vi "UserVars-Get Bernoulli Function.vi"(0 "Expr in":string, 11 "error in (no error)":errorcluster) -> (6 "X":dbl[](array[numeric]), 8 "PDF":dbl[](array[numeric]), 10 "Ref Pts":dbl[](array[numeric]), 15 "error out":errorcluster)   [LabVIEW 2020]
uses:
  <vilib>/Analysis/1siggen.llb/Ramp Pattern by Samples.vi
  <vilib>/regexp/Match Regular Expression.xnode
  <vilib>/Analysis/NI_AALBase.lvlib
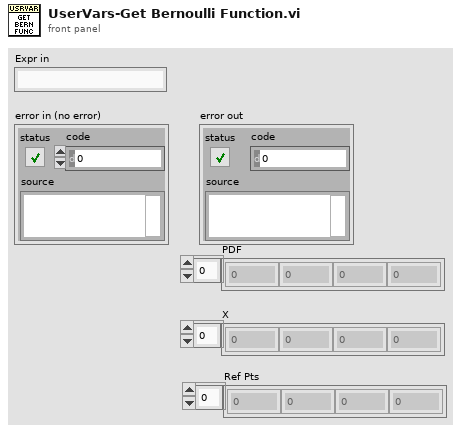
[diagram p1: front panel]
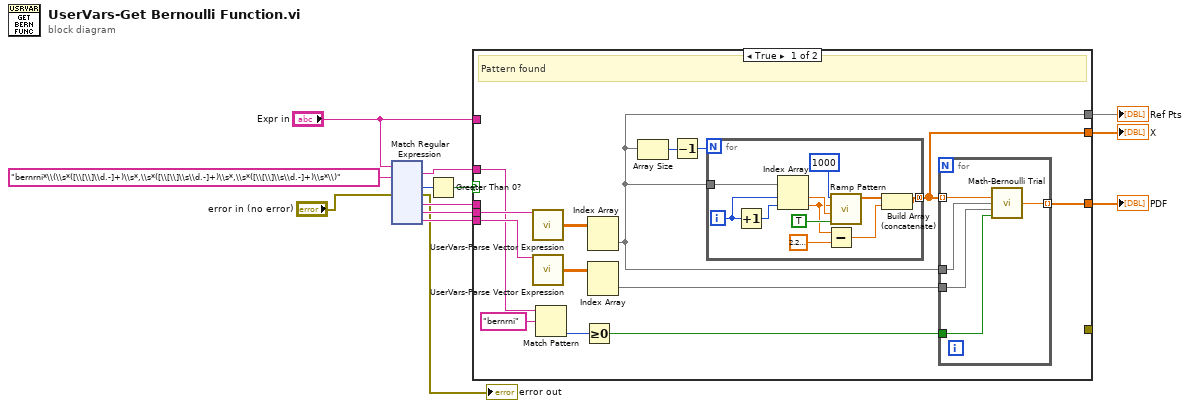
[diagram p0: block diagram]
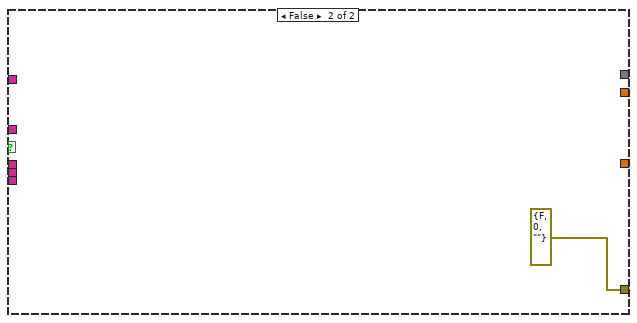
[diagram p2: hidden frame]
diagram:
  n1 = xnode "Match Regular Expression"("input string"="Expr in", "regular expression"="bernrni*\\(\\s*([\\[\\]\\d.-]+)\\s*,\\s*([\\[\\]\\s\\d.-]+)\\s*,\\s*([\\[\\]\\s\\d.-]+)\\s*\\)" ("String"), "error in"="error in (no error)") -> ("whole match"=w10:string, "offset past match"=w11:i32, "error out"=→"error out":errorcluster, "submatch 1"=w9:string, "submatch 2"=w8:string, "submatch 3"=w6:string)  [unwired: 3 in, 2 out]
  n2 = Greater Than 0?(x=w11) -> (x > 0?=w7:bool)
  n3 = case shown="True" w7 {
    tunnel: "Expr in" -> [_ _]
    tunnel: w10 -> [w17 _]
    tunnel: w9 -> [_ _]
    tunnel: w8 -> [w27 _]
    tunnel: w6 -> [w26 _]
    tunnel: [w20 _] -> w4
    tunnel: [_ errorcluster {"status"=FALSE, "code"=0, "source"=""} ("error constant")] -> _
    tunnel: [w21 _] -> w2
    tunnel: [w18 _] -> w1
    frame True {
      # "Pattern found"
      n4 = call "UserVars-Parse Vector Expression.vi"("Expression In"=w27) -> ("values"=w25:dbl[][])  [unwired: 11 in, 3 out]
      n5 = call "UserVars-Parse Vector Expression.vi"("Expression In"=w26) -> ("values"=w24:dbl[][])  [unwired: 11 in, 3 out]
      n6 = Match Pattern(string=w17, regular expression="bernrni") -> (offset past match=w15:i32)  [unwired: 1 in, 3 out]
      n7 = Greater Or Equal To 0?(x=w15) -> (x >= 0?=w14:bool)
      n8 = Index Array(array=w25) -> (element=w20:dbl[])  [unwired: 2 in]
      n9 = Index Array(array=w24) -> (element=w19:dbl[])  [unwired: 2 in]
      n10 = Array Size(array=w20) -> (size(s)=w23:i32)
      n11 = Decrement(x=w23) -> (x-1=w22:i32)
      n12 = for {
        N: w22 -> [_]
        tunnel: w20 -> [w43]
        tunnel: [w37] -> w21 mode=concatenating
        i -> [w42]
        n13 = Increment(x=w42) -> (x+1=w41:i32)
        n14 = Index Array(array=w43, index #1=w42, index #2=w41) -> (element #1=w36:dbl, element #2=w33:dbl)
        n15 = Subtract(x=w33, y=2.220446049250313e-16) -> (x-y=w35:dbl)
        n16 = call-poly <vilib>:"Ramp Pattern.vi"("exclude end?"=TRUE, "start"=w36, "end"=w33, "samples"=1000) -> ("Ramp Pattern"=w38:dbl[])  [unwired: 6 in, 1 out]
        n17 = Build Array (concatenate)(w38, w35) -> (w37:dbl[])
      }
      n18 = for {
        tunnel: w21 -> [w32] mode=indexing
        tunnel: w20 -> [w31]
        tunnel: w19 -> [w30]
        tunnel: [w29] -> w18 mode=indexing
        tunnel: w14 -> [w28]
        n19 = call "Math-Bernoulli Trial.vi"("U"=w32, "X"=w31, "PofX"=w30, "interpolate"=w28) -> ("Prob"=w29:dbl)  [unwired: 10 in, 1 out]
      }
    }
    frame False {
    }
  }
  "PDF" <- w1
  "X" <- w2
  "Ref Pts" <- w4
